vi "DataFileName(SubVI).vi"(4 "error in (no error)":errorcluster, 5 "Date":string, 6 "Segment":string, 7 "CPR":string) -> (0 "error out":errorcluster, 2 "Relative path":path, 3 "Path":path)   [LabVIEW 2013, in "main.lvlib"]
uses:
  main.lvlib
  Globals/DataPathGlobalVariable.vi
  <userlib>/_OpenG.lib/file/file.llb/File Exists - Scalar__ogtk.vi
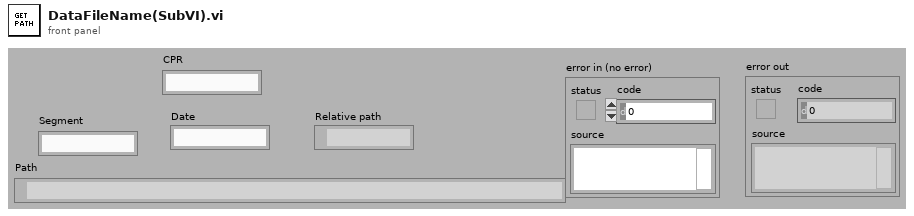
[diagram p1: front panel]
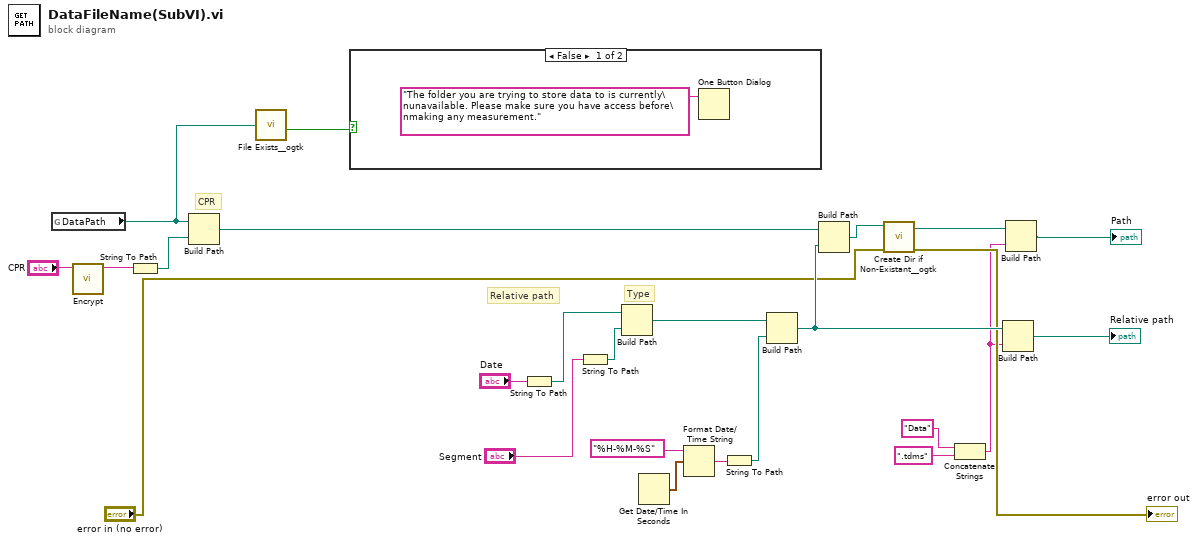
[diagram p0: block diagram]
diagram:
  # "Relative path"
  # "Type"
  # "CPR"
  n1 = global read "DataPathGlobalVariable.vi" "DataPath"() -> (w3:path)
  n2 = call "Encrypt.vi"("Input"="CPR") -> ("Output"=w24:string)  [unwired: 10 in]
  n3 = String To Path(string=w24) -> (path=w25:path)
  n4 = Build Path(base path=w3, name or relative path=w25) -> (appended path=w10:path)
  n5 = call-poly <userlib>:"File Exists__ogtk.vi"("file path"=w3) -> ("exists"=w13:bool)  [unwired: 6 in, 1 out]
  n6 = case shown="False" w13 {
    frame False {
      n7 = One Button Dialog(message="The folder you are trying to store data to is currently\nunavailable. Please make sure you have access before\nmaking any measurement.") -> ()  [unwired: 1 in, 1 out]
    }
    frame True {
    }
  }
  n8 = String To Path(string="Date") -> (path=w12:path)
  n9 = String To Path(string="Segment") -> (path=w22:path)
  n10 = Build Path(base path=w12, name or relative path=w22) -> (appended path=w16:path)
  n11 = Get Date/Time In Seconds() -> (seconds since 1Jan1904=w19:timestamp)
  n12 = Format Date/Time String(time format string (%c)="%H-%M-%S", seconds (now)=w19) -> (date/time string=w18:string)  [unwired: 1 in]
  n13 = String To Path(string=w18) -> (path=w17:path)
  n14 = Build Path(base path=w16, name or relative path=w17) -> (appended path=w9:path)
  n15 = Build Path(base path=w10, name or relative path=w9) -> (appended path=w8:path)
  n16 = call <userlib>:"Create Dir if Non-Existant__ogtk.vi"("error in (no error)"="error in (no error)", "Directory Path"=w8) -> ("error out"=→"error out":errorcluster, "dup Directory Path"=w5:path)  [unwired: 7 in, 1 out]
  n17 = Concatenate Strings("Data", ".tdms" ("string")) -> (w4:string)
  n18 = Build Path(base path=w9, name or relative path=w4) -> (appended path=→"Relative path":path)
  n19 = Build Path(base path=w5, name or relative path=w4) -> (appended path=→"Path":path)
